vi "CheckData(SubVI).vi"(8 "Error In":errorcluster, 11 "String in":string) -> (0 "Error Out":errorcluster)   [LabVIEW 2018]
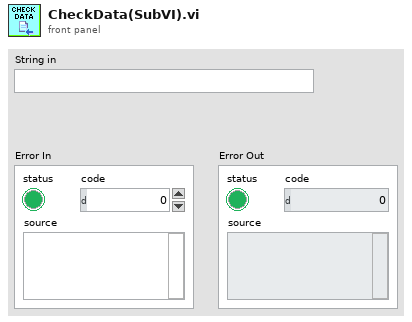
[diagram p1: front panel]
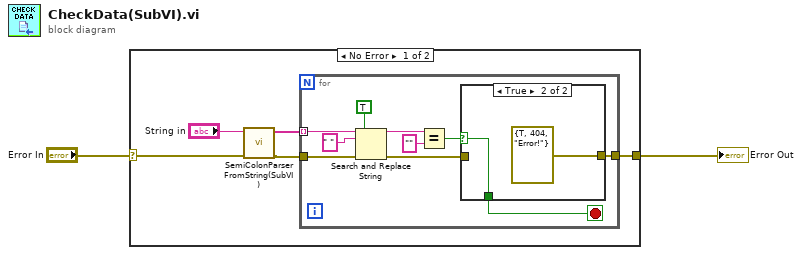
[diagram p0: block diagram]
diagram:
  n1 = case shown="No Error" "Error In" {
    selector: "Error In" -> [w6 w21]
    tunnel: [w4 w21] -> w1
    frame No Error {
      n2 = call "SemiColonParserFromString(SubVI).vi"("Error In"=w6, "String In"="String in") -> ("Error Out"=w3:errorcluster, "String Array Out"=w5:string[])  [unwired: 8 in]
      n3 = for {
        tunnel: w5 -> [w12] mode=indexing
        tunnel: [w15] -> w4
        tunnel: w3 -> [w11]
        stop <- w9 stop-if-true
        n4 = Search and Replace String(replace all?=TRUE ("replace all? (F)"), input string=w12, search string=" ", error in=w11) -> (result string=w10:string, error out=w8:errorcluster)  [unwired: 4 in, 2 out]
        n5 = Equal?(x=w10, y="") -> (x = y?=w16:bool)
        n6 = case shown="True" w16 {
          selector: w16 -> [_ w19]
          tunnel: [w18 errorcluster {"status"=TRUE, "code"=404, "source"="Error!"} ("error IO")] -> w15
          tunnel: [_ w19] -> w9
          tunnel: w8 -> [w18 _]
          frame False {
          }
          frame True {
          }
        }
      }
    }
    frame Error {
    }
  }
  "Error Out" <- w1
